vi "Close Instrument.vi"(7 "Go Local (\"@LOC\")":bool, 8 "error in (no error)":errorcluster, 11 "Agilent DSO1000 in":refnum<class "Agilent DSO1000.lvclass">) -> (0 "error out":errorcluster, 3 "Agilent DSO1000 out":refnum<class "Agilent DSO1000.lvclass">)   [LabVIEW 2020, in "Agilent DSO1000.lvclass"]
uses:
  Agilent DSO1000.lvclass
  C:/Sandbox/RF Bench/Source Code/WiSpry Test Framework/Instruments/Instrument.lvclass
  Instrument.lvclass/Instrument.ctl
  Instrument.lvclass
  <instrlib>/Agilent DSO1000 Series/Agilent DSO1000 Series.lvlib
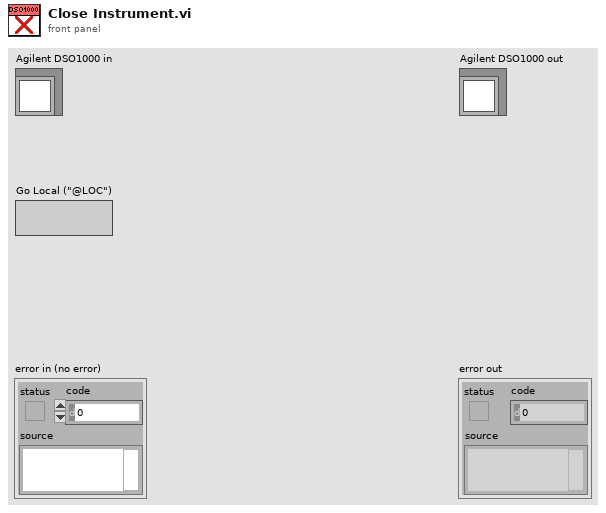
[diagram p1: front panel]
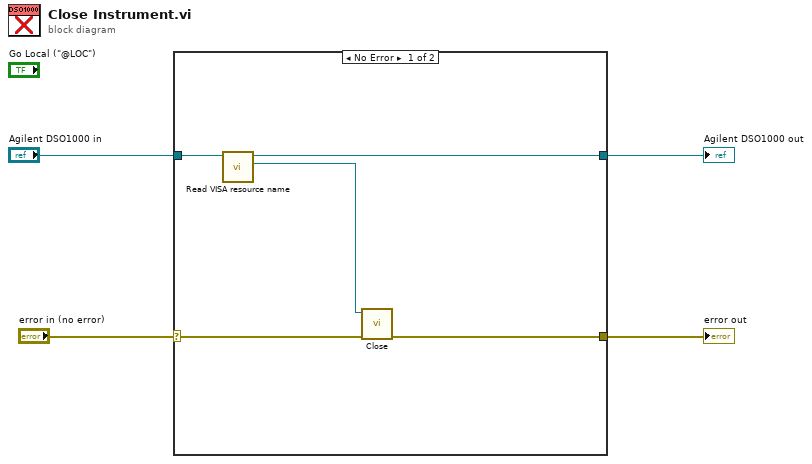
[diagram p0: block diagram]
diagram:
  n1 = case shown="No Error" "error in (no error)" {
    selector: "error in (no error)" -> [w7 w11]
    tunnel: [w6 w11] -> w3
    tunnel: [w8 w10] -> w2
    tunnel: "Agilent DSO1000 in" -> [w9 w10]
    frame No Error {
      n2 = call "Read VISA resource name.vi"("Instrument in"=w9) -> ("VISA resource name"=w5:refnum<visa-resource-name>, "Instrument out"=w8:refnum<class "Agilent DSO1000.lvclass">)  [unwired: 9 in]
      n3 = call <instrlib>:"Close.vi"("error in (no error)"=w7, "VISA resource name"=w5) -> ("error out"=w6:errorcluster)  [unwired: 9 in]
    }
    frame Error {
    }
  }
  "error out" <- w3
  "Agilent DSO1000 out" <- w2
